vi "confic screen.vi"(9 "User Name":string="User Type", 10 "Path":path, 11 "vi path":path) -> (0 "error out":errorcluster, 3 "VI out":refnum<vi>)   [LabVIEW 2015]
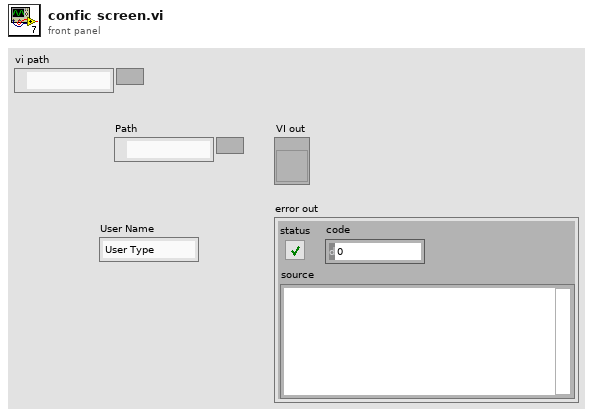
[diagram p1: front panel]
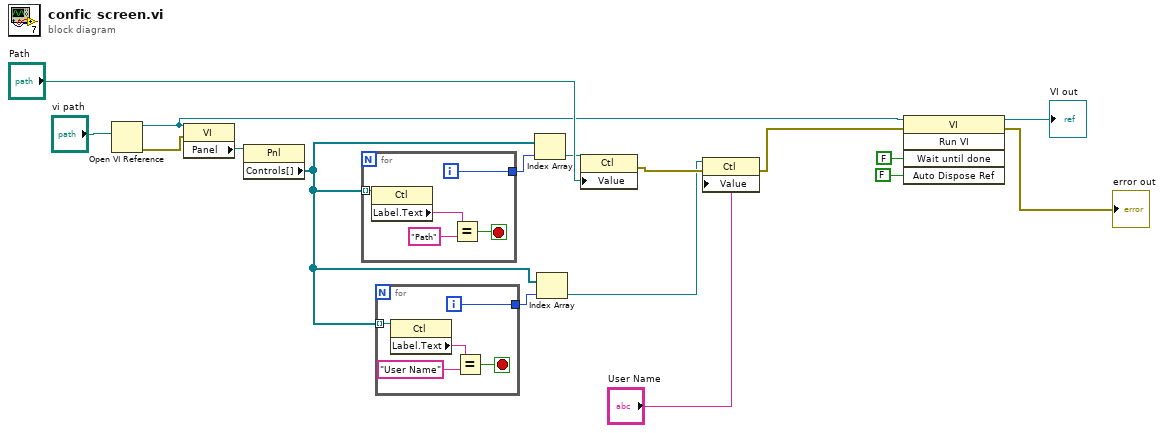
[diagram p0: block diagram]
diagram:
  n1 = Open VI Reference(vi path="vi path") -> (vi reference=w15:refnum<vi>, error out=w13:errorcluster)  [unwired: 5 in]
  n2 = property class="VI"(reference=w15, error in=w13) -> ("Panel"=w14:refnum<vi>)  [unwired: 2 out]
  n3 = property class="Pnl"(reference=w14) -> ("Controls[]"=w6:refnum<vi>[])  [unwired: 1 in, 2 out]
  n4 = for {
    tunnel: w6 -> [w22] mode=indexing
    tunnel: [w18] -> w16
    i -> [w18]
    stop <- w19 stop-if-true
    n5 = property class="Ctl"(reference=w22) -> ("Label.Text"=w21:string)  [unwired: 1 in, 2 out]
    n6 = Equal?(x=w21, y="Path") -> (x = y?=w19:bool)
  }
  n7 = for {
    tunnel: w6 -> [w27] mode=indexing
    tunnel: [w23] -> w7
    i -> [w23]
    stop <- w24 stop-if-true
    n8 = property class="Ctl"(reference=w27) -> ("Label.Text"=w26:string)  [unwired: 1 in, 2 out]
    n9 = Equal?(x=w26, y="User Name") -> (x = y?=w24:bool)
  }
  n10 = Index Array(array=w6, index=w16) -> (element=w4:refnum<vi>)
  n11 = Index Array(array=w6, index=w7) -> (element=w3:refnum<vi>)
  n12 = property class="Ctl"(reference=w4, "Value"="Path") -> (error out=w5:errorcluster)  [unwired: 1 in, 1 out]
  n13 = property class="Ctl"(reference=w3, error in=w5, "Value"="User Name") -> (error out=w1:errorcluster)  [unwired: 1 out]
  n14 = invoke class="VI" method="Run VI"(reference=w15, error in=w1, "Wait until done"=FALSE, "Auto Dispose Ref"=FALSE ("Auto Dispose Reference")) -> (reference out=→"VI out":refnum<vi>, error out=→"error out":errorcluster)  [unwired: 1 in, 3 out]
